vi "Plot Default Sine Graph.vi"() -> ()   [LabVIEW 2020]
panel:
  out "Data":dbl[](array[numeric])
  out "Waveform Graph":dbl[](graph)
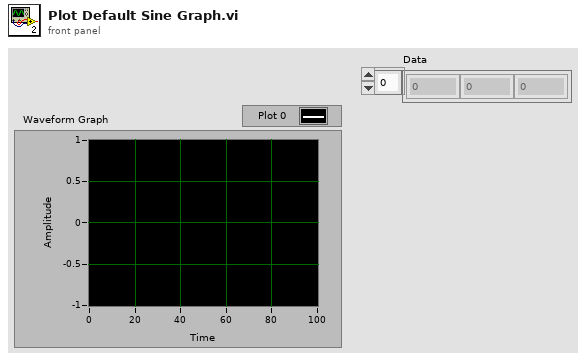
[diagram p1: front panel]
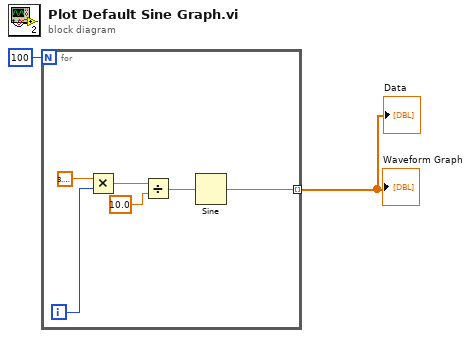
[diagram p0: block diagram]
diagram:
  n1 = for {
    N: 100 -> [_]
    tunnel: [w3] -> w1 mode=indexing
    i -> [w8]
    n2 = Multiply(x=3.141592653589793, y=w8) -> (x*y=w6:dbl)
    n3 = Divide(x=w6, y=10.0 ("x")) -> (x/y=w4:dbl)
    n4 = Sine(x=w4) -> (sin(x)=w3:dbl)
  }
  "Waveform Graph" <- w1
  "Data" <- w1
